vi "TW Adjust Library Icons.vi"(6 "Debug":bool, 7 "Overlay Icon":refnum<class "Icon.lvclass">, 8 "error in":errorcluster, 10 "Library Names":string[](array[string])=["TemplatePlugin.lvclass", "TemplatePlugin.lvlib", "TemplateCommon.lvlib", "TemplateWrapper.lvlib"], 11 "Library Map in":map{string, refnum<vi>}(c390)) -> (0 "error out":errorcluster caption="error in", 3 "Library Map out":map{string, refnum<vi>}(c390), 4 "Result for debugging":cluster{"Name":string, picture[]}[](array[cluster]))   [LabVIEW 2021, in "LV Scripting Utilities.lvlib"]
uses:
  LV Scripting Utilities.lvlib
  <vilib>/LabVIEW Icon API/LabVIEW Icon API.lvlib
  <vilib>/LabVIEW Icon API/lv_icon/Classes/Icon/Icon.lvclass
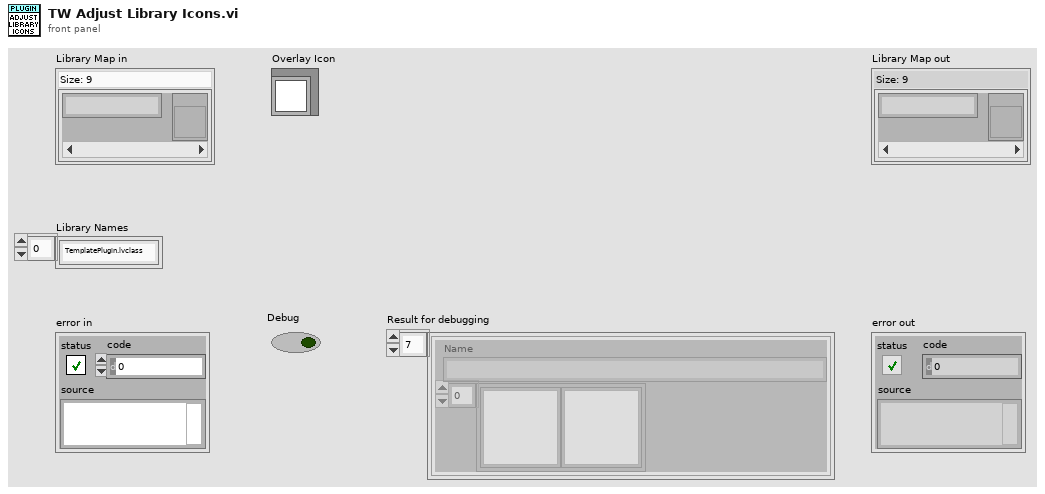
[diagram p1: front panel]
types:
  T1 = typedef "imagedata.ctl" = cluster{"image type":i32, "image depth":i32, "image":u8[], "mask":u8[], "colors":u32[], "Rectangle":cluster{"left":i16, "top":i16, "right":i16, "bottom":i16}}
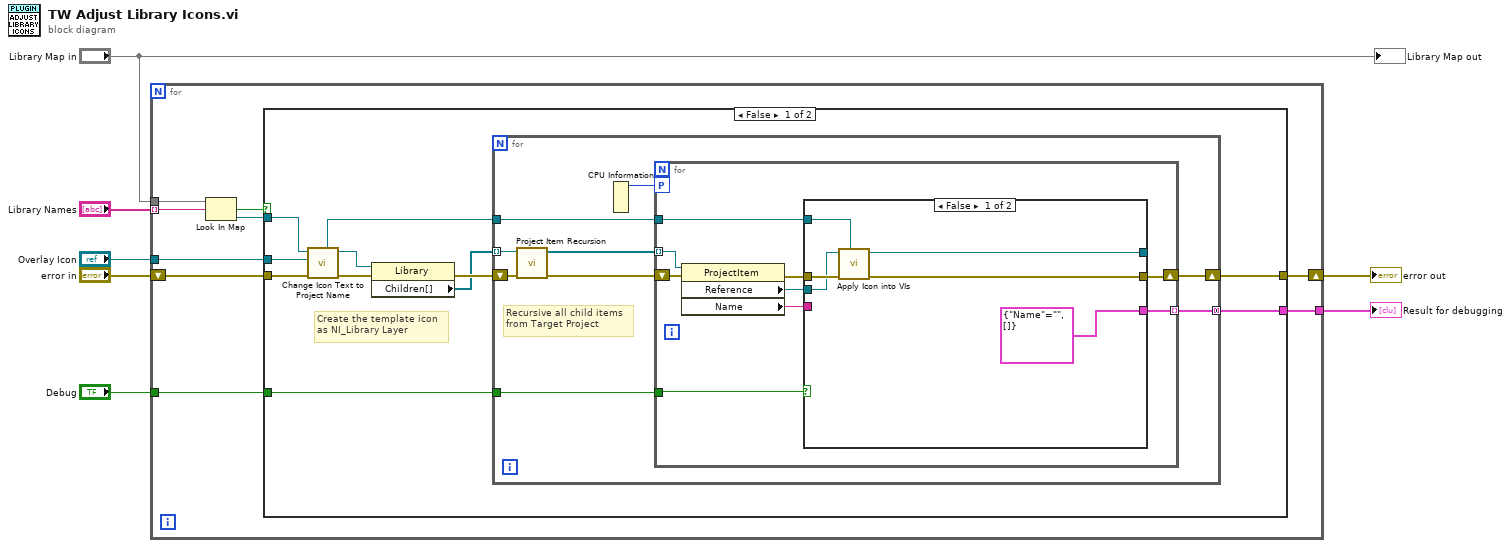
[diagram p0: block diagram]
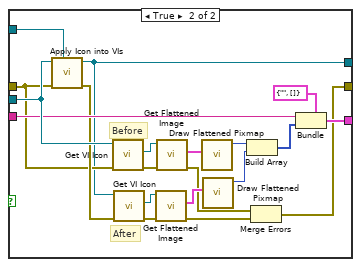
[diagram p2: hidden frame]
diagram:
  n1 = for {
    tunnel: "Library Map in" -> [w16]
    tunnel: "Debug" -> [w13]
    tunnel: "Overlay Icon" -> [w10]
    tunnel: [w9] -> w2
    shift-right: [w11] -> w4
    shift-left: "error in" -> [w12]
    tunnel: "Library Names" -> [w8] mode=indexing
    n2 = Look In Map(map=w16, key=w8) -> (key not found?=w15:bool, value=w14:refnum<vi>)  [unwired: 1 in]
    n3 = case shown="False" w15 {
      tunnel: w14 -> [w27 _]
      tunnel: w13 -> [w24 _]
      tunnel: w12 -> [w23 w72]
      tunnel: [w22 w72] -> w11
      tunnel: w10 -> [w20 _]
      tunnel: [w18 _] -> w9
      frame False {
        # "Create the template icon\nas NI_Library Layer"
        n4 = call "Change Icon Text to Project Name.vi"("error in"=w23, "Overlay Icon"=w20, "Lvclass Ref in"=w27) -> ("error out"=w26:errorcluster, "Lvclass Ref out"=w21:refnum<vi>, "Layer.lvclass out"=w17:refnum<class "Layer.lvclass">)  [unwired: 5 in, 1 out]
        n5 = property class="Library"(reference=w21, error in=w26) -> (error out=w25:errorcluster, "Children[]"=w19:refnum<vi>[])  [unwired: 1 out]
        n6 = for {
          tunnel: w19 -> [w36] mode=indexing
          tunnel: [w34] -> w18 mode=concatenating
          tunnel: w17 -> [w32]
          tunnel: w24 -> [w31]
          shift-right: [w28] -> w22
          shift-left: w25 -> [w30]
          # "Recursive all child items\nfrom Target Project"
          n7 = call "Project Item Recursion.vi"("error in"=w30, "TargetItem in"=w36) -> ("error out"=w33:errorcluster, "TargetItem out"=w35:refnum<vi>[])  [unwired: 8 in]
          n8 = CPU Information() -> (4:w29:i32)  [unwired: 3 out]
          n9 = for {
            tunnel: w35 -> [w45] mode=indexing
            tunnel: [w43] -> w34 mode=indexing
            tunnel: w32 -> [w38]
            workers-P: w29 -> [_]
            tunnel: w31 -> [w39]
            shift-right: [w37] -> w28
            shift-left: w33 -> [w44]
            n10 = property class="ProjectItem"(reference=w45, error in=w44) -> (error out=w40:errorcluster, "Reference"=w42:refnum<vi>, "Name"=w41:string)  [unwired: 1 out]
            n11 = case shown="False" w39 {
              tunnel: [cluster{"Name":string, picture[]} {"Name"="", []} ("cluster") w71] -> w43
              tunnel: w42 -> [w46 w70]
              tunnel: w41 -> [_ w69]
              tunnel: [w49 w67] -> w37
              tunnel: w40 -> [w51 w54]
              tunnel: w38 -> [w50 w53]
              tunnel: [w47 w52] -> _
              frame False {
                n12 = call "Apply Icon into VIs.vi"("Substitute Layer"=w50, "error in"=w51, "VI in"=w46) -> ("error out"=w49:errorcluster, "VI Refnum out"=w47:refnum<vi>)  [unwired: 7 in]
              }
              frame True {
                # "After"
                # "Before"
                n13 = call "Apply Icon into VIs.vi"("Substitute Layer"=w53, "error in"=w54, "VI in"=w70) -> ("error out"=w68:errorcluster, "VI Refnum out"=w52:refnum<vi>)  [unwired: 7 in]
                n14 = call <vilib>:"Get VI Icon.vi"("error in (no error)"=w54, "VI Refnum in"=w70) -> ("error out"=w58:errorcluster, "Icon"=w64:refnum<class "Icon.lvclass">)  [unwired: 7 in, 1 out]
                n15 = call <vilib>:"Get VI Icon.vi"("error in (no error)"=w68, "VI Refnum in"=w52) -> ("error out"=w57:errorcluster, "Icon"=w66:refnum<class "Icon.lvclass">)  [unwired: 7 in, 1 out]
                n16 = call <vilib>:"Get Flattened Image.vi"("error in (no error)"=w57, "lv_icon.lvlib:Icon.lvclass in"=w66) -> ("error out"=w55:errorcluster, "Color Image"=w65:T1)  [unwired: 6 in, 2 out]
                n17 = call <vilib>:"Get Flattened Image.vi"("error in (no error)"=w58, "lv_icon.lvlib:Icon.lvclass in"=w64) -> ("error out"=w56:errorcluster, "Color Image"=w63:T1)  [unwired: 6 in, 2 out]
                n18 = call <vilib>:"Draw Flattened Pixmap.vi"("image data"=w63) -> ("new picture"=w62:picture)  [unwired: 8 in]
                n19 = call <vilib>:"Draw Flattened Pixmap.vi"("image data"=w65) -> ("new picture"=w61:picture)  [unwired: 8 in]
                n20 = Build Array(w62, w61) -> (w60:picture[])
                n21 = Merge Errors(w56, w55) -> (w67:errorcluster)
                n22 = Bundle(cluster=cluster{"Name":string, picture[]} {"Name"="", []}, "Name"=w69, w60) -> (w71:cluster{"Name":string, picture[]})
              }
            }
          }
        }
      }
      frame True {
        # "Could add error that expected library not found"
      }
    }
  }
  "error out" <- w4
  "Result for debugging" <- w2
  "Library Map out" <- "Library Map in"
